vi "binary_get_metadata.vi"(8 "error in":errorcluster, 10 "all in one package in":T1={"memory structure"={"length of metadata [byte]"=5, "length of page [byte]"=2048, "length of measurement data on page [byte]"=2028, "length of dataset [byte]"=6}, "actigraph settings"={"sampling frequency [Hz]"=0.0, "measurement interval [± g]"=0, "high precision?"=FALSE, "number of pages"=0, "rate code"=0, "range code"=0, "id"=0}, "time informations"={"starting time"=timestamp(0 s since 1904-01-01), "ending time"=timestamp(0 s since 1904-01-01), "dt[s]"=0.0, "sampling rate [Hz]"=0.0, "length"=0.0}, "measurement data"={"number of samples per axis"=0, "timestamp array"=[], "offset array"=[], "x, y, z axis data"=[], "normalised magnitude of acceleartion vectors"={"t0"=timestamp(0 s since 1904-01-01), "dt"=1.0, "Y"=[]}, "calibration coefficients"={"Sx"=0.0, "Ox"=0.0, "Sy"=0.0, "Oy"=0.0, "Sz"=0.0, "Oz"=0.0}, "statistics"={"mean of x axis acceleration"=0.0, "standard devation of x axis acceleration"=0.0, "mean of y axis acceleration"=0.0, "standard devation of y axis acceleration"=0.0, "mean of z axis acceleration"=0.0, "standard devation of z axis acceleration"=0.0, "mean of normalised magnitude of acceleration"=0.0, "standard devation of normalised magnitude of acceleration"=0.0}, "battery voltage"={"t0"=timestamp(0 s since 1904-01-01), "dt"=1.0, "Y"=[]}, "magnitude of acceleartion vectors"={"t0"=timestamp(0 s since 1904-01-01), "dt"=1.0, "Y"=[]}}} {"measurement data"."calibration coefficients"."Oz" format="%#_12g"; "measurement data"."calibration coefficients"."Sz" format="%#_12g"; "measurement data"."calibration coefficients"."Oy" format="%#_12g"; "measurement data"."calibration coefficients"."Sy" format="%#_12g"; "measurement data"."calibration coefficients"."Ox" format="%#_12g"; "measurement data"."calibration coefficients"."Sx" format="%#_12g"; "time informations"."length" format="%<%H:%M:%S%3u>t"; "actigraph settings"."id" format="%02d"; "actigraph settings"."range code" format="%02x"; "actigraph settings"."rate code" format="%02x"}, 11 "binary data w/ calibration coefficients":u8[](array[numeric])) -> (0 "error out":errorcluster, 2 "all in one package out":T1={"memory structure"={"length of metadata [byte]"=5, "length of page [byte]"=2048, "length of measurement data on page [byte]"=2028, "length of dataset [byte]"=6}, "actigraph settings"={"sampling frequency [Hz]"=0.0, "measurement interval [± g]"=0, "high precision?"=FALSE, "number of pages"=0, "rate code"=0, "range code"=0, "id"=0}, "time informations"={"starting time"=timestamp(0 s since 1904-01-01), "ending time"=timestamp(0 s since 1904-01-01), "dt[s]"=0.0, "sampling rate [Hz]"=0.0, "length"=0.0}, "measurement data"={"number of samples per axis"=0, "timestamp array"=[], "offset array"=[], "x, y, z axis data"=[], "normalised magnitude of acceleartion vectors"={"t0"=timestamp(0 s since 1904-01-01), "dt"=1.0, "Y"=[]}, "calibration coefficients"={"Sx"=0.0, "Ox"=0.0, "Sy"=0.0, "Oy"=0.0, "Sz"=0.0, "Oz"=0.0}, "statistics"={"mean of x axis acceleration"=0.0, "standard devation of x axis acceleration"=0.0, "mean of y axis acceleration"=0.0, "standard devation of y axis acceleration"=0.0, "mean of z axis acceleration"=0.0, "standard devation of z axis acceleration"=0.0, "mean of normalised magnitude of acceleration"=0.0, "standard devation of normalised magnitude of acceleration"=0.0}, "battery voltage"={"t0"=timestamp(0 s since 1904-01-01), "dt"=1.0, "Y"=[]}, "magnitude of acceleartion vectors"={"t0"=timestamp(0 s since 1904-01-01), "dt"=1.0, "Y"=[]}}} {"measurement data"."calibration coefficients"."Oz" format="%#_12g"; "measurement data"."calibration coefficients"."Sz" format="%#_12g"; "measurement data"."calibration coefficients"."Oy" format="%#_12g"; "measurement data"."calibration coefficients"."Sy" format="%#_12g"; "measurement data"."calibration coefficients"."Ox" format="%#_12g"; "measurement data"."calibration coefficients"."Sx" format="%#_12g"; "time informations"."length" format="%<%H:%M:%S%3u>t"; "actigraph settings"."id" format="%02d"; "actigraph settings"."range code" format="%02x"; "actigraph settings"."rate code" format="%02x"}, 3 "pages":u8[](array[numeric]))   [LabVIEW 2020]
uses:
  Controls/control_all_in_one_package.ctl
  Controls/control_memory_structure.ctl
  Controls/control_measurement_settings.ctl
  Controls/control_time_informations.ctl
  Controls/control_measurement_data.ctl
  Controls/control_calibration_coefficients.ctl
  Controls/control_statistics.ctl
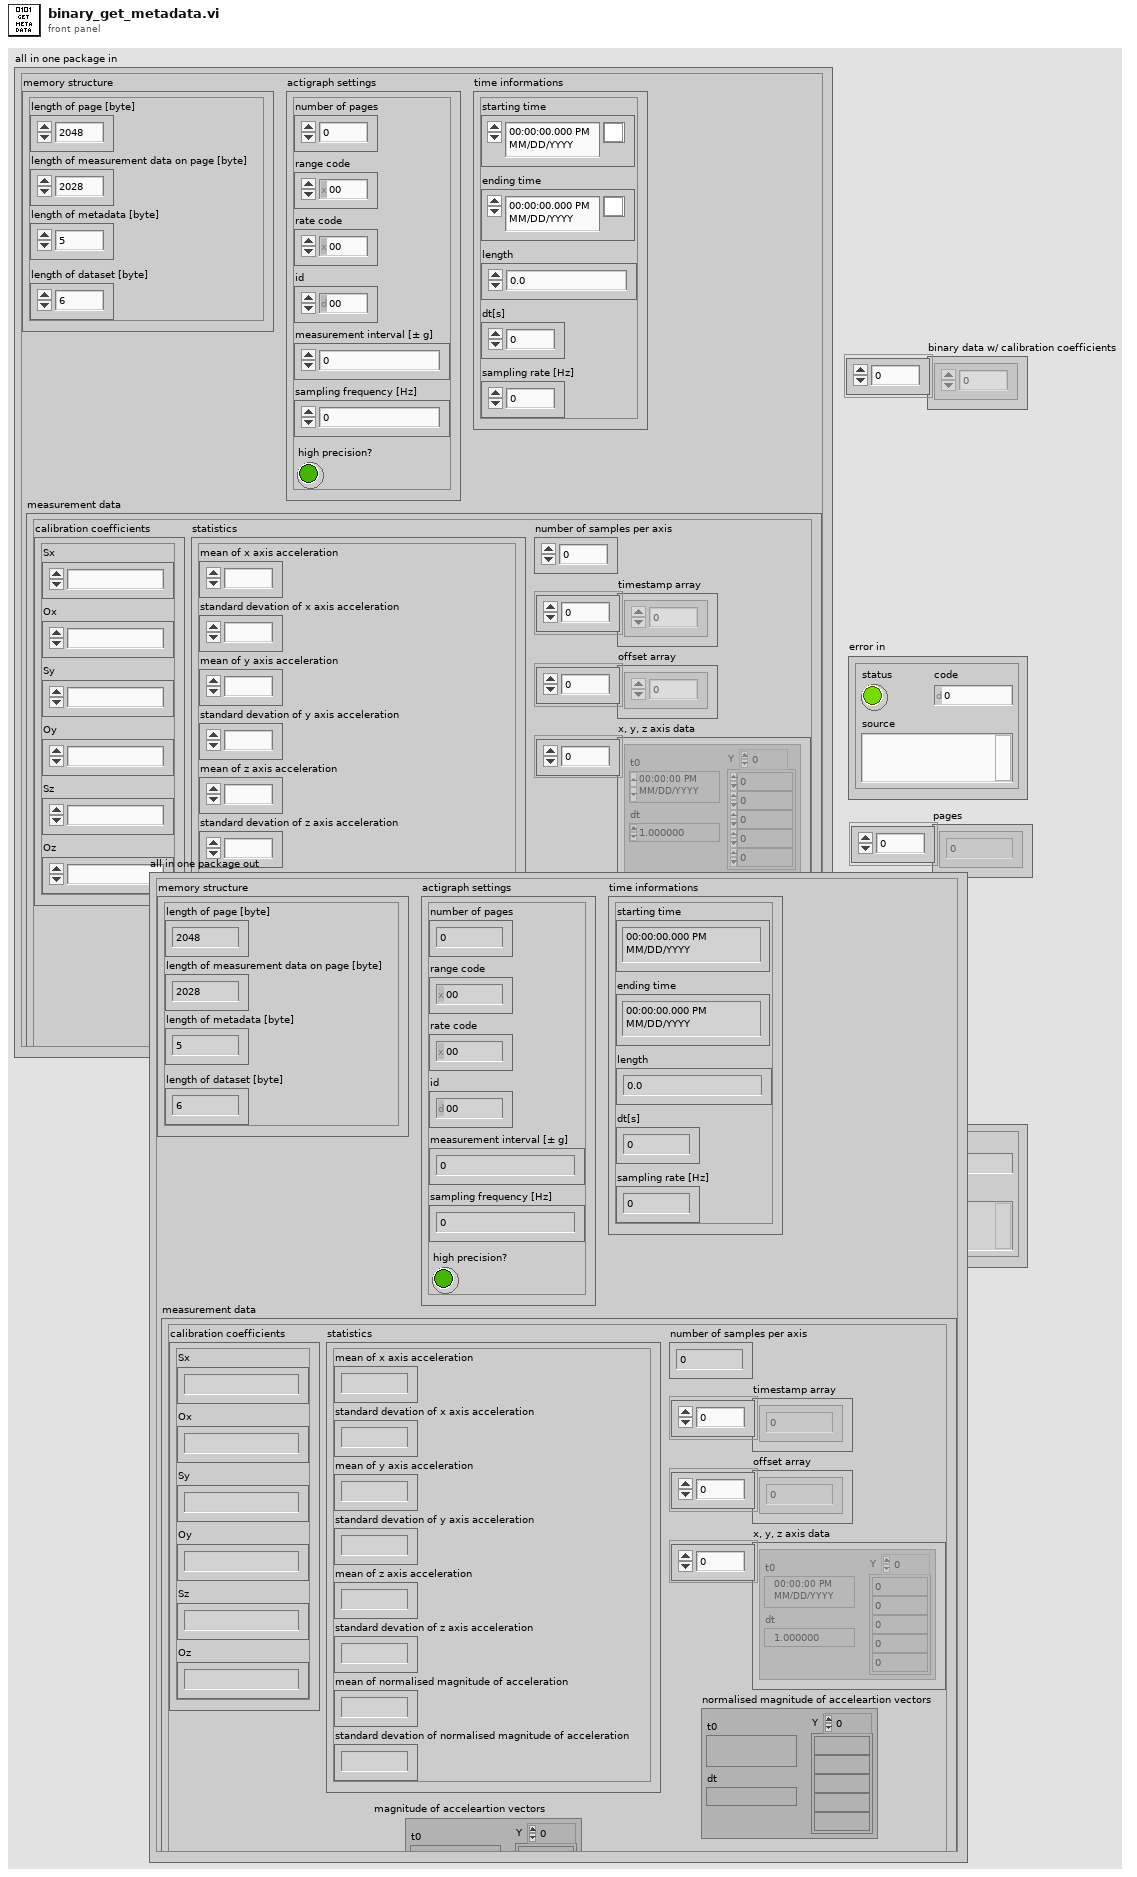
[diagram p1: front panel]
types:
  T1 = typedef "control_all_in_one_package.ctl" = cluster{"memory structure":T2, "actigraph settings":T3, "time informations":T4, "measurement data":T5}
  T2 = typedef "control_memory_structure.ctl" = cluster{"length of metadata [byte]":i32, "length of page [byte]":i32, "length of measurement data on page [byte]":i32, "length of dataset [byte]":i32}
  T3 = typedef "control_measurement_settings.ctl" = cluster{"sampling frequency [Hz]":dbl, "measurement interval [± g]":i32, "high precision?":bool, "number of pages":i32, "rate code":i32, "range code":i32, "id":i32}
  T4 = typedef "control_time_informations.ctl" = cluster{"starting time":timestamp, "ending time":timestamp, "dt[s]":dbl, "sampling rate [Hz]":dbl, "length":dbl}
  T5 = typedef "control_measurement_data.ctl" = cluster{"number of samples per axis":i32, "timestamp array":dbl[], "offset array":dbl[], "x, y, z axis data":waveform(dbl)[], "normalised magnitude of acceleartion vectors":waveform(dbl), "calibration coefficients":T6, "statistics":T7, "battery voltage":waveform(dbl), "magnitude of acceleartion vectors":waveform(dbl)}
  T6 = typedef "control_calibration_coefficients.ctl" = cluster{"Sx":dbl, "Ox":dbl, "Sy":dbl, "Oy":dbl, "Sz":dbl, "Oz":dbl}
  T7 = typedef "control_statistics.ctl" = cluster{"mean of x axis acceleration":dbl, "standard devation of x axis acceleration":dbl, "mean of y axis acceleration":dbl, "standard devation of y axis acceleration":dbl, "mean of z axis acceleration":dbl, "standard devation of z axis acceleration":dbl, "mean of normalised magnitude of acceleration":dbl, "standard devation of normalised magnitude of acceleration":dbl}
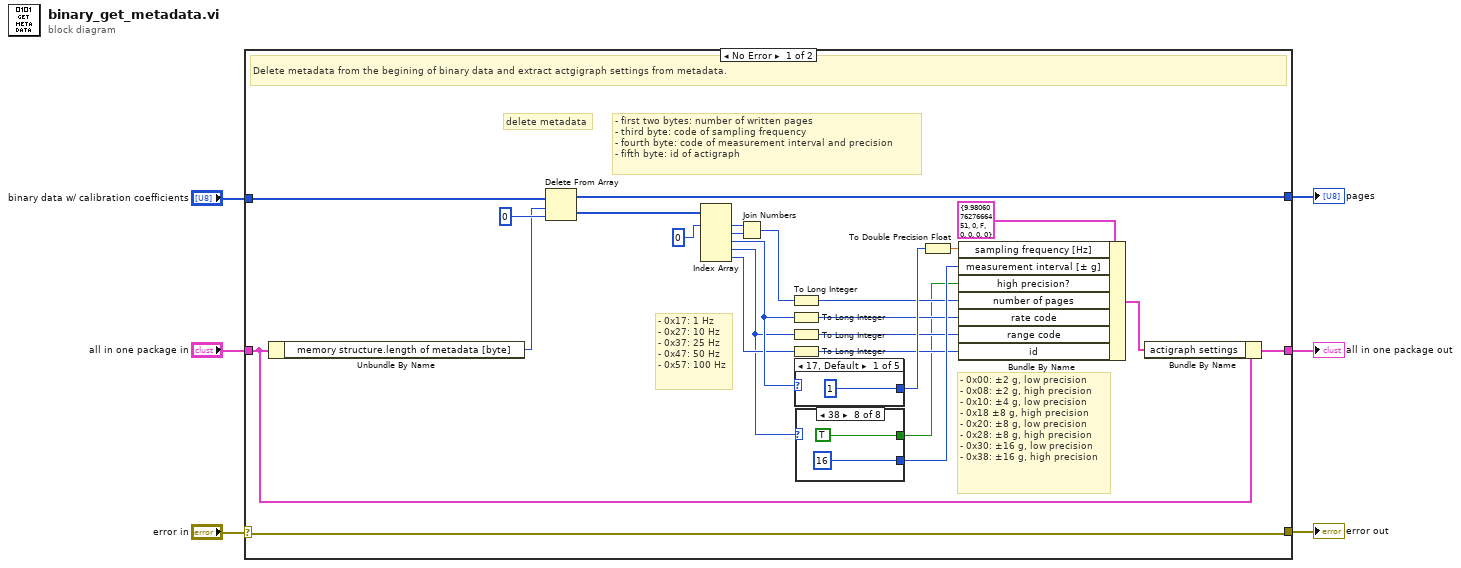
[diagram p0: block diagram]
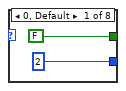
[diagram p2: hidden frame]
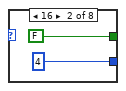
[diagram p3: hidden frame]
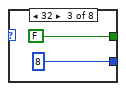
[diagram p4: hidden frame]
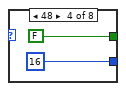
[diagram p5: hidden frame]
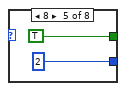
[diagram p6: hidden frame]
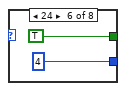
[diagram p7: hidden frame]
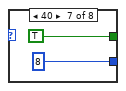
[diagram p8: hidden frame]
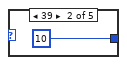
[diagram p9: hidden frame]
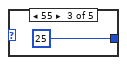
[diagram p10: hidden frame]
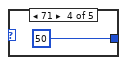
[diagram p11: hidden frame]
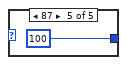
[diagram p12: hidden frame]
diagram:
  n1 = case shown="No Error" "error in" {
    selector: "error in" -> [w29 w55]
    tunnel: [w29 w55] -> w5
    tunnel: "binary data w/ calibration coefficients" -> [w25 w53]
    tunnel: [w22 w53] -> w3
    tunnel: "all in one package in" -> [w12 w54]
    tunnel: [w10 w54] -> w1
    frame No Error {
      # "- 0x00: ±2 g, low precision\n- 0x08: ±2 g, high precision\n- 0x10: ±4 g, low precision\n- 0x18 ±8 g, high precision\n- 0x20: ±8 g, low precision\n- 0x28: ±8 g, high precision\n- 0x30: ±16 g, low precision\n- 0x38: ±16 g, high precision"
      # "- 0x17: 1 Hz\n- 0x27: 10 Hz\n- 0x37: 25 Hz\n- 0x47: 50 Hz\n- 0x57: 100 Hz"
      # "- first two bytes: number of written pages\n- third byte: code of sampling frequency\n- fourth byte: code of measurement interval and precision\n- fifth byte: id of actigraph"
      # "delete metadata"
      # "Delete metadata from the begining of binary data and extract actgigraph settings from metadata."
      n2 = Unbundle By Name(w12) -> ("memory structure.length of metadata [byte]"=w13:i32)
      n3 = Delete From Array(array=w25, length=w13, index=0) -> (deleted portion=w23:u8[], array with subset deleted=w22:u8[])
      n4 = Index Array(array=w23, index #1=0 ("index")) -> (element #1=w31:u8, element #2=w30:u8, element #3=w27:u8, element #4=w8:u8, element #5=w26:u8)  [unwired: 4 in]
      n5 = Join Numbers(hi=w31, lo=w30) -> ((hi.lo)=w28:u16)
      n6 = To Long Integer(number=w28) -> (32bit integer=w18:i32)
      n7 = To Long Integer(number=w27) -> (32bit integer=w17:i32)
      n8 = To Long Integer(number=w8) -> (32bit integer=w16:i32)
      n9 = To Long Integer(number=w26) -> (32bit integer=w15:i32)
      n10 = case shown="17, Default" w27 {
        tunnel: [1 10 25 50 100] -> w21
        frame 23, Default {
        }
        frame 39 {
        }
        frame 55 {
        }
        frame 71 {
        }
        frame 87 {
        }
      }
      n11 = case shown="38" w8 {
        tunnel: [2 4 8 16 2 4 8 16] -> w19
        tunnel: [FALSE FALSE FALSE FALSE TRUE TRUE TRUE TRUE] -> w9
        frame 0, Default {
        }
        frame 16 {
        }
        frame 32 {
        }
        frame 48 {
        }
        frame 8 {
        }
        frame 24 {
        }
        frame 40 {
        }
        frame 56 {
        }
      }
      n12 = To Double Precision Float(number=w21) -> (double precision float=w20:dbl)
      n13 = Bundle By Name(cluster=T3 {"sampling frequency [Hz]"=9.980607627666451, "measurement interval [± g]"=0, "high precision?"=FALSE, "number of pages"=0, "rate code"=0, "range code"=0, "id"=0} ("measurement settings"), "sampling frequency [Hz]"=w20, "measurement interval [± g]"=w19, "high precision?"=w9, "number of pages"=w18, "rate code"=w17, "range code"=w16, "id"=w15) -> (w11:T3)
      n14 = Bundle By Name(cluster=w12, "actigraph settings"=w11) -> (w10:T1)
    }
    frame Error {
    }
  }
  "error out" <- w5
  "pages" <- w3
  "all in one package out" <- w1
